vi "SLSC Diagram Window.vi"() -> ()   [LabVIEW 2019, in "SLSC-12201 DIO System Explorer.lvlib"]
uses:
  SLSC-12201 DIO System Explorer.lvlib
  <vilib>/picture/picture.llb/imagedata.ctl
panel:
  out "2D Picture":picture
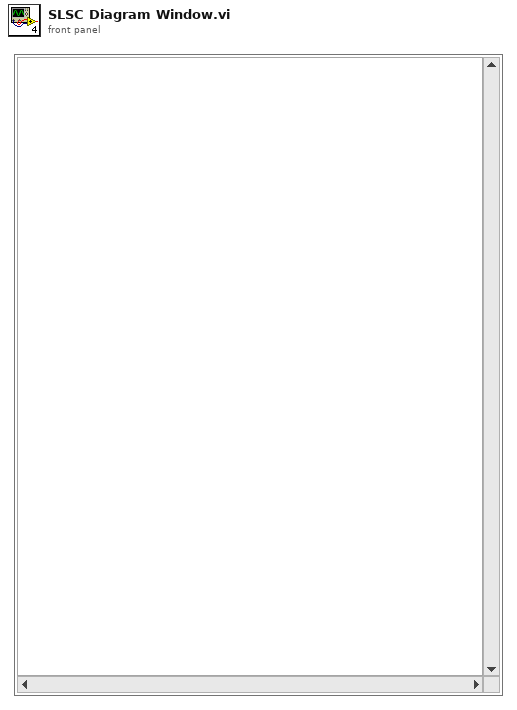
[diagram p1: front panel]
types:
  T1 = typedef "imagedata.ctl" = cluster{"image type":i32, "image depth":i32, "image":u8[], "mask":u8[], "colors":u32[], "Rectangle":cluster{"left":i16, "top":i16, "right":i16, "bottom":i16}}
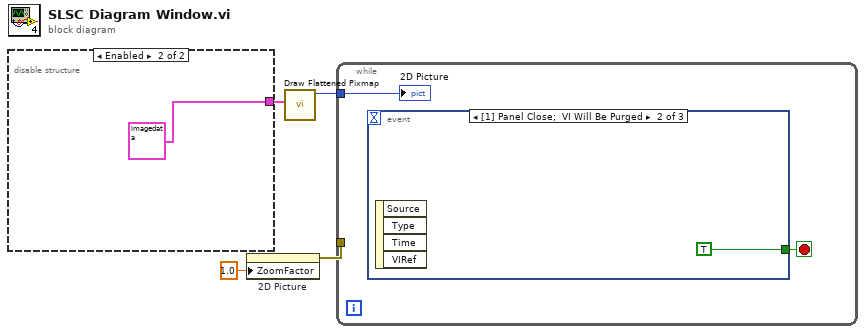
[diagram p0: block diagram]
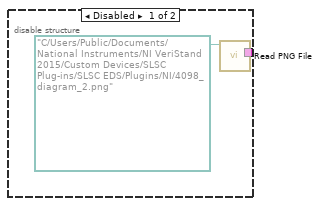
[diagram p2: hidden frame]
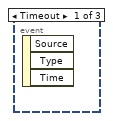
[diagram p3: hidden frame]
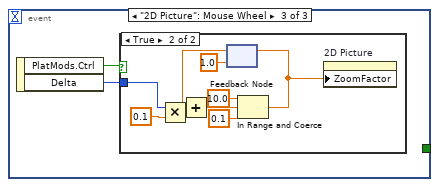
[diagram p4: hidden frame]
diagram:
  n1 = disable-structure shown="Enabled" {
    disable-tunnel: [w5 T1 {"image type"=0, "image depth"=32, "image"=array[1096868 elements], "mask"=array[34664 elements], "colors"=[], "Rectangle"={"left"=0, "top"=0, "right"=443, "bottom"=619}} ("image data")] -> w1
    frame Disabled {
      n2 = call <vilib>:"Read PNG File.vi"("path to PNG file"=path "C:/Users/Public/Documents/National Instruments/NI VeriStand 2015/Custom Devices/SLSC Plug-ins/SLSC EDS/Plugins/NI/4098_diagram_2.png") -> ("image data"=w5:T1)  [unwired: 8 in, 2 out]
    }
    frame Enabled {
    }
  }
  n3 = property on="2D Picture" class="Pict"("ZoomFactor"=sgl 1.0 ("Zoom Factor")) -> (error out=w2:errorcluster)  [unwired: 2 in, 1 out]
  n4 = call <vilib>:"Draw Flattened Pixmap.vi"("image data"=w1) -> ("new picture"=w4:picture)  [unwired: 8 in]
  n5 = while {
    tunnel: w4 -> [w8]
    tunnel: w2 -> [_]
    stop <- w9 stop-if-true
    n6 = event shown="[1] Panel Close;  VI Will Be Purged" {
      selector: _ -> [_ _ _]
      dyn-events: _ -> [_ _ _]
      timeout: _ -> [_ _ _]
      tunnel: [_ TRUE _] -> w9
      event Timeout {
        n7 = event-data() -> ()  [unwired: 1 in, 3 out]
      }
      event Panel Close; event #0x24 {
        n8 = event-data() -> ()  [unwired: 1 in, 4 out]
      }
      event "2D Picture": Mouse Wheel {
        n9 = event-data() -> ("PlatMods.Ctrl"=w11:bool, "Delta"=w12:i32)  [unwired: 1 in]
        n10 = case shown="True" w11 {
          tunnel: w12 -> [_ w17]
          frame False {
          }
          frame True {
            n11 = Multiply(x=w17, y=0.1) -> (x*y=w20:dbl)
            n12 = feedback #1(1.0 ("upper limit")) -> (w18:dbl)
            n13 = Add(x=w18, y=w20) -> (x+y=w19:dbl)
            n14 = In Range and Coerce(upper limit=10.0, x=w19, lower limit=0.1) -> (coerced(x)=w16:dbl)  [unwired: 1 out]
            n15 = feedback-in #1(w16) -> ()
            n16 = property on="2D Picture" class="Pict"("ZoomFactor"=w16) -> ()  [unwired: 2 in, 2 out]
          }
        }
      }
    }
    "2D Picture" <- w8
  }
